vi "Transition Timeout Check.vi"(6 "Start Time":u32, 9 "Timeout limit":u16, 10 "Current State in":T1, 11 "Modified Array of states in":T1[](array[typedef])) -> (0 "Status Message":string, 1 "millisecond timer value out":u32, 2 "Next State":T1, 3 "Modified Array of states out":T1[](array[typedef]))   [LabVIEW 2016]
doc: "Tranision Timeout Check takes the current state, modified array of states, timeout limit, and start time to: \n\n(1) determine if process has timed out\n(2) what state to progress to next, and \n(3) what the current status message should be."
uses:
  SC2 states.ctl
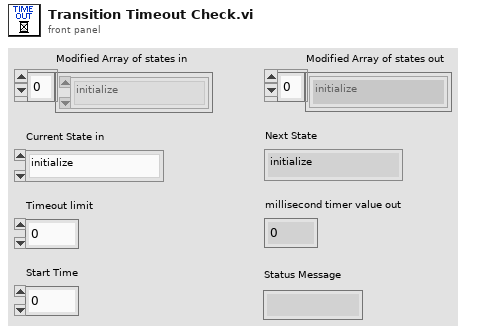
[diagram p1: front panel]
types:
  T1 = typedef "SC2 states.ctl" = enum16{"initialize", "wait", "change sample start", "change sample", "check position", "rotate wheel", "sample change complete", "sample rod up", "sample rod down", "retract rod in", "retract rod out", "insert rod in", "insert rod out", "wheel GV open", "wheel GV close", "ion source GV open", "ion source GV close", "vent source", "pump source", "Shutdown"}
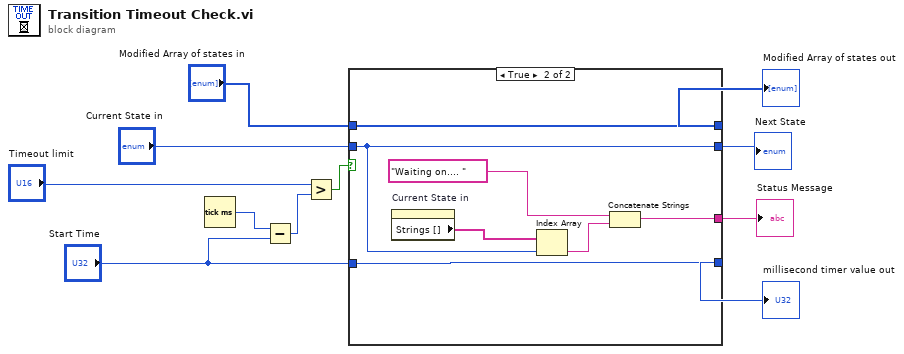
[diagram p0: block diagram]
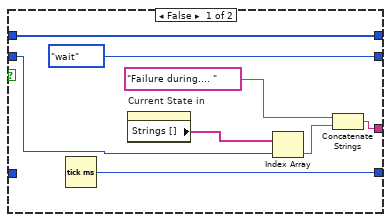
[diagram p2: hidden frame]
diagram:
  n1 = Tick Count (ms)() -> (millisecond timer value=w2:u32)
  n2 = Subtract(x=w2, y="Start Time") -> (x-y=w3:u32)
  n3 = Greater?(x="Timeout limit", y=w3) -> (0:w4:bool)
  n4 = case shown="True" w4 {
    tunnel: "Current State in" -> [w13 w23]
    tunnel: [SC2_states."wait" ("Current State") w23] -> w6
    tunnel: "Modified Array of states in" -> [w18 w26]
    tunnel: [w18 w26] -> w8
    tunnel: "Start Time" -> [_ w25]
    tunnel: [w19 w25] -> w10
    tunnel: [w12 w20] -> w1
    frame False {
      n5 = Tick Count (ms)() -> (millisecond timer value=w19:u32)
      n6 = property on="Current State in" class="Enum (strict)"() -> ("Strings []"=w16:string[])  [unwired: 2 in, 2 out]
      n7 = Index Array(array=w16, index=w13) -> (element=w15:string)
      n8 = Concatenate Strings("Failure during.... ", w15) -> (w12:string)
    }
    frame True {
      n9 = property on="Current State in" class="Enum (strict)"() -> ("Strings []"=w24:string[])  [unwired: 2 in, 2 out]
      n10 = Index Array(array=w24, index=w23) -> (element=w22:string)
      n11 = Concatenate Strings("Waiting on.... ", w22) -> (w20:string)
    }
  }
  "millisecond timer value out" <- w10
  "Modified Array of states out" <- w8
  "Next State" <- w6
  "Status Message" <- w1
